vi "Check what current project is.vi"(5 "Project Name":string="I2C_Core") -> (0 "Project":string, 1 "ProjectName":T1=enum."SPIM", 2 "Input = Current Project,\nor project not defined?":bool)   [LabVIEW 2012]
doc: "This .vi returns the current project. The input can be connected to determine if the current project is the same as the input string. To perform this logic, the .vi searches the ProjectName project variable for the input string."
uses:
  File IO/Config/ProjectName enum.ctl
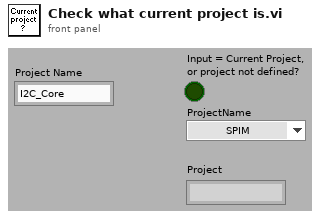
[diagram p1: front panel]
types:
  T1 = typedef "ProjectName enum.ctl" = enum16{"V-SIM", "SPIM", "TEMca2", "undefined", "I2C_Core"}
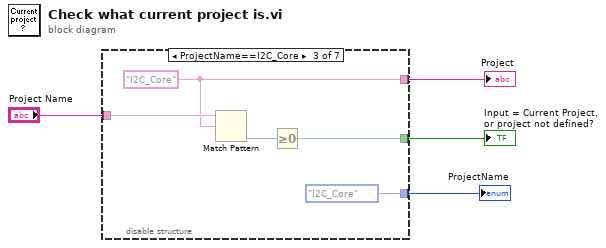
[diagram p0: block diagram]
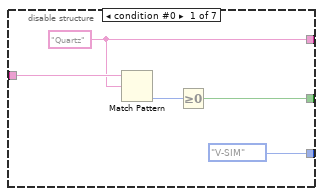
[diagram p2: hidden frame]
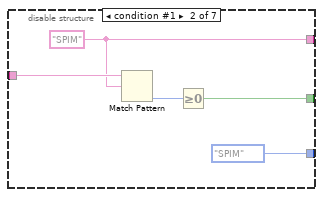
[diagram p3: hidden frame]
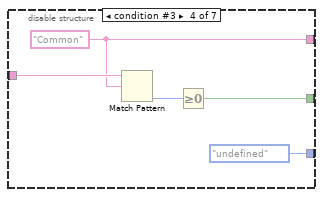
[diagram p4: hidden frame]
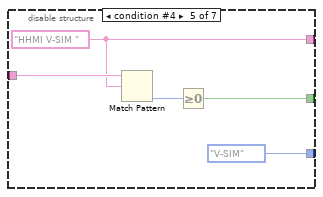
[diagram p5: hidden frame]
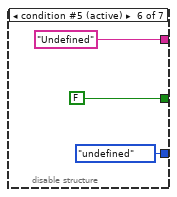
[diagram p6: hidden frame]
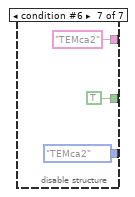
[diagram p7: hidden frame]
diagram:
  n1 = disable-structure shown="ProjectName==I2C_Core" {
    disable-tunnel: "Project Name" -> [w9 w14 w19 w24 w29 _ _]
    disable-tunnel: [w7 w12 w17 w22 w27 FALSE TRUE ("Input = Current Project,\nor project not defined?")] -> w4
    disable-tunnel: [w6 w11 w16 w21 w26 "Undefined" ("Project") "TEMca2" ("Project")] -> w2
    disable-tunnel: [ProjectName_enum."V-SIM" ("ProjectName") ProjectName_enum."SPIM" ("ProjectName") ProjectName_enum."I2C_Core" ("ProjectName") ProjectName_enum."undefined" ("ProjectName") ProjectName_enum."V-SIM" ("ProjectName") ProjectName_enum."undefined" ("ProjectName") ProjectName_enum."TEMca2" ("ProjectName")] -> w1
    frame condition #0 {
      w6 = "Quartz" ("Name")
      n2 = Match Pattern(string=w9, regular expression=w6) -> (offset past match=w8:i32)  [unwired: 4 out]
      n3 = Greater Or Equal To 0?(x=w8) -> (x >= 0?=w7:bool)
    }
    frame condition #1 {
      w11 = "SPIM" ("Name")
      n4 = Match Pattern(string=w14, regular expression=w11) -> (offset past match=w13:i32)  [unwired: 4 out]
      n5 = Greater Or Equal To 0?(x=w13) -> (x >= 0?=w12:bool)
    }
    frame condition #2 {
      w16 = "I2C_Core" ("Name")
      n6 = Match Pattern(string=w19, regular expression=w16) -> (offset past match=w18:i32)  [unwired: 4 out]
      n7 = Greater Or Equal To 0?(x=w18) -> (x >= 0?=w17:bool)
    }
    frame condition #3 {
      w21 = "Common" ("Name")
      n8 = Match Pattern(string=w24, regular expression=w21) -> (offset past match=w23:i32)  [unwired: 4 out]
      n9 = Greater Or Equal To 0?(x=w23) -> (x >= 0?=w22:bool)
    }
    frame condition #4 {
      w26 = "HHMI V-SIM " ("Name")
      n10 = Match Pattern(string=w29, regular expression=w26) -> (offset past match=w28:i32)  [unwired: 4 out]
      n11 = Greater Or Equal To 0?(x=w28) -> (x >= 0?=w27:bool)
    }
    frame condition #5 (active) {
    }
    frame condition #6 {
    }
  }
  "Input = Current Project,\nor project not defined?" <- w4
  "Project" <- w2
  "ProjectName" <- w1
